vi "Set ReadRate.vi"(10 "ReadRate":dbl format="%#_g Hz", 11 "Worker in":refnum<class "Communicator Worker.lvclass">) -> (3 "Worker out":refnum<class "Communicator Worker.lvclass">)   [LabVIEW 2025, in "Communicator Worker.lvlib" / "Communicator Worker.lvclass"]
uses:
  Communicator Worker.lvclass
  Communicator Worker.lvclass/Communicator Worker.ctl
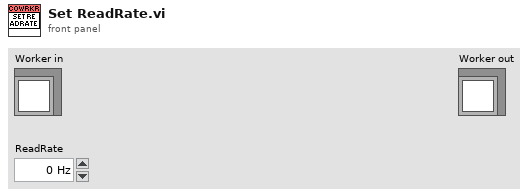
[diagram p1: front panel]
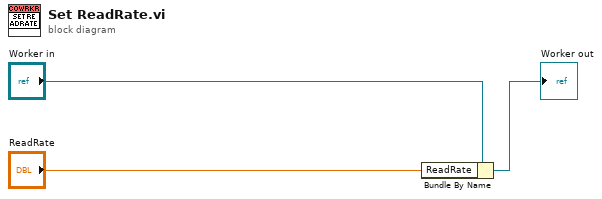
[diagram p0: block diagram]
diagram:
  n1 = Bundle By Name(cluster="Worker in", "ReadRate"="ReadRate") -> (→"Worker out":refnum<class "Communicator Worker.lvclass">)
